vi "Create Visualizer.vi"(8 "error in (no error)":errorcluster, 10 "Front Panel Bounds":T1) -> (0 "error out":errorcluster, 3 "Visualizer ID":T2)   [LabVIEW 2010, in "Visualizer.lvlib"]
doc: "Creates a new visualizer window and returns the visualizer ID for that window. Use the Front Panel Bounds input to specify the display size of the panel."
uses:
  Visualizer.lvlib
  Visualizer Type ID.ctl
  <vilib>/Utility/miscctls.llb/LVRectTypeDef.ctl
  Display.vi
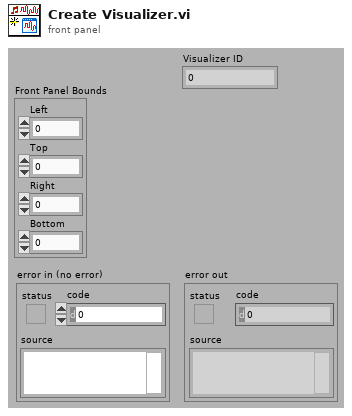
[diagram p1: front panel]
types:
  T1 = typedef "LVRectTypeDef.ctl" = cluster{"Left":i16, "Top":i16, "Right":i16, "Bottom":i16}
  T2 = typedef "Visualizer.lvlib/Visualizer Type ID.ctl" = u32
  T3 = cluster{"Left":bool, "Top":bool, "Right":bool, "Bottom":bool}
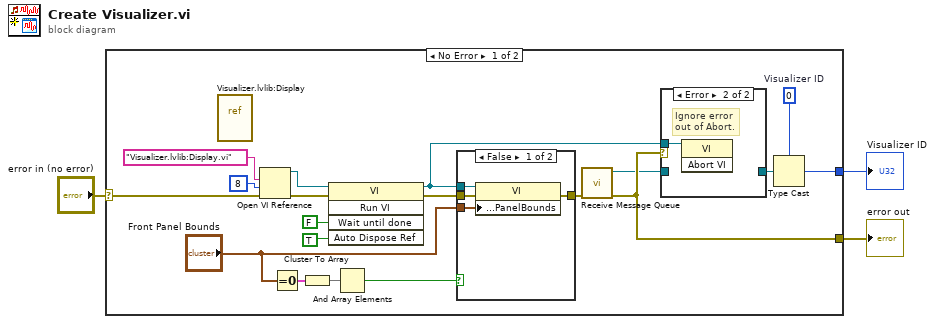
[diagram p0: block diagram]
diagram:
  n1 = case shown="No Error" "error in (no error)" {
    selector: "error in (no error)" -> [w21 w30]
    tunnel: [w15 w30] -> w2
    tunnel: [w16 _] -> w1
    frame No Error {
      w12 = T2 0  # Visualizer ID
      n2 = vi-ref "Visualizer.lvlib:Display.vi"() -> ()  [unwired: 1 out]
      n3 = Open VI Reference(vi path="Visualizer.lvlib:Display.vi", options=8, error in (no error)=w21) -> (vi reference=w20:refnum<vi>, error out=w19:errorcluster)  [unwired: 3 in]
      n4 = Equal To 0?(x="Front Panel Bounds") -> (x = 0?=w6:T3)
      n5 = Cluster To Array(cluster=w6) -> (array=w5:bool[])
      n6 = invoke class="VI" method="Run VI"(reference=w20, error in=w19, "Wait until done"=FALSE ("Wait Until Done"), "Auto Dispose Ref"=TRUE ("Auto Dispose Reference")) -> (reference out=w10:refnum<vi>, error out=w11:errorcluster)  [unwired: 1 in, 3 out]
      n7 = And Array Elements(Boolean array=w5) -> (logical AND=w4:bool)
      n8 = case shown="False" w4 {
        tunnel: w11 -> [w26 w27]
        tunnel: w10 -> [w25 _]
        tunnel: [w24 w27] -> w9
        tunnel: "Front Panel Bounds" -> [w23 _]
        frame False {
          n9 = property class="VI"(reference=w25, error in=w26, "Front Panel.PanelBounds"=w23) -> (error out=w24:errorcluster)  [unwired: 1 out]
        }
        frame True {
        }
      }
      n10 = call "Receive Message Queue.vi"("error in (no error)"=w9) -> ("error out"=w15:errorcluster, "queue out"=w14:refnum<queue>)  [unwired: 9 in]
      n11 = case shown="Error" w15 {
        tunnel: w10 -> [_ w29]
        tunnel: w14 -> [w28 _]
        tunnel: [w28 _] -> w13
        frame No Error {
        }
        frame Error {
          # "Ignore error\nout of Abort."
          n12 = invoke class="VI" method="Abort VI"(reference=w29) -> ()  [unwired: 2 in, 3 out]
        }
      }
      n13 = Type Cast(type=w12, x=w13) -> (*(type *) &x=w16:T2)
    }
    frame Error {
    }
  }
  "error out" <- w2
  "Visualizer ID" <- w1
